vi "Config.vi"() -> ()   [LabVIEW 2010, in "DCP551.lvlib"]
uses:
  DCP551.lvlib
panel:
  in  "Tab Control":T1(tab)
  in  "Read Registers":T2
  in  "Start":bool
  in  "Stop":bool
  in  "Exit":bool
  in  "Server Status":string
  in  "Segment 1 to 99":T3(array[cluster])
  in  "Segment 0":T4={"Start"=enum."Non PV start", "Cycle data"=0, "Pattern link data"=0, "Tag data"="12345678"}
  in  "File ID":string="1"
  in  "Read File":bool
  in  "Write File":bool
  in  "Config":bool
  in  "Serial Config":T5={"串口选择"="COM1", "通讯速率"=9600, "超时时间"=200, "数据位长"=8, "奇偶校验"=enum."Even", "停止位长"=10, "握手控制"=0, "字符结束"=TRUE, "结束字符"=10, "仪器地址"=1} {"结束字符" format="%.0x"; "握手控制" items=["None", "XON/XOFF", "RTS/CTS", "XON/XOFF & RTS/CTS", "DTR/DSR", "XON/XOFF & DTR/DSR"]; "停止位长" items=["1.0"=10, "1.5"=15, "2.0"=20]; "数据位长" min=5 max=8 step=1}
  in  "Write Registers":T6
  in  "RUN":bool
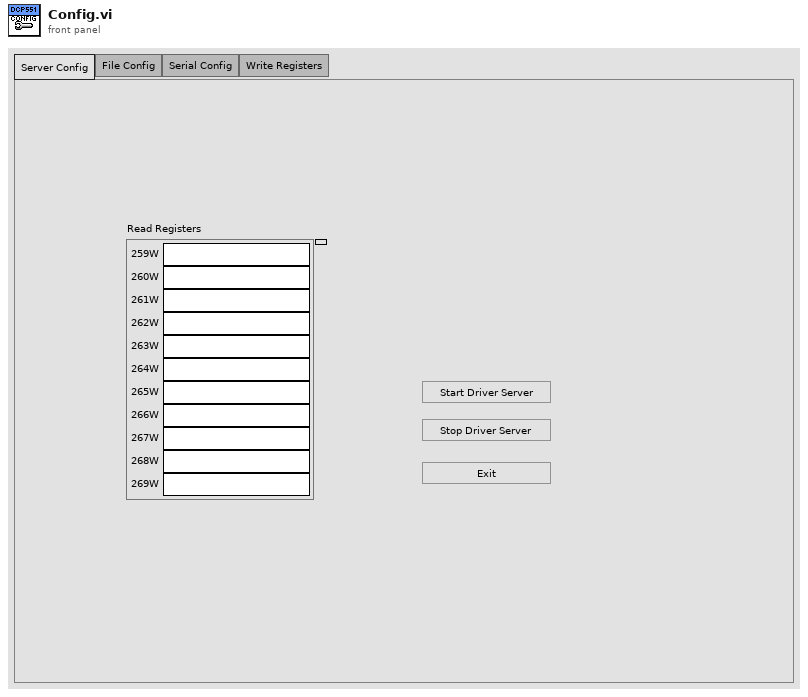
[diagram p1: front panel]
types:
  T1 = enum32{"Server Config", "File Config", "Serial Config", "Write Registers"}
  T2 = cluster{"259W":string, "260W":string, "261W":string, "262W":string, "263W":string, "264W":string, "265W":string, "266W":string, "267W":string, "268W":string, "269W":string}
  T3 = cluster{"SP":dbl, "Time":cluster{"Type":enum16{"Time Data", "delta Dtada", "SP Data"}, "Data":i32}, "EV1 to 16":cluster{"Event 1st data":i32, "Event 2nd data":i32}[], "Output limiter group data":i32, "PID group data":i32, "Repeat return segment data":i32, "Repeat data":i32, "G. soak type data":enum16{"G. soak setting is not provided", "Segment start point", "Segment end point", "Total segment"}, "G. soak width data":i32, "PV shift data":i32}[]
  T4 = cluster{"Start":enum16{"Non PV start", "Upward PV tart", "Downward PV start", "Either upward of downward PV start"}, "Cycle data":i32, "Pattern link data":i32, "Tag data":string}
  T5 = cluster{"串口选择":refnum<visa-resource-name>, "通讯速率":u32, "超时时间":u32, "数据位长":u16, "奇偶校验":enum16{"None", "Odd", "Even", "Mark", "Space"}, "停止位长":u16, "握手控制":u16, "字符结束":bool, "结束字符":u8, "仪器地址":u32}
  T6 = cluster{"261W":string, "262W":string, "263W":string, "264W":string, "265W":string}
  T7 = enum32{"invalid app kind", "Development System", "Run Time System", "Student Edition", "Embedded LabVIEW", "Evaluation", "Custom"}
  T8 = enum32{"Invalid", "Standard", "Closed", "Hidden", "Minimized", "Maximized"}
  T9 = cluster{"Core":cluster{"Current VI Reference":refnum<vi>, "Close Panel on Exit?":bool}, "Your Boolean data":bool, "Your string data":string}
  T10 = cluster{"Current VI Reference":refnum<vi>, "Close Panel on Exit?":bool}
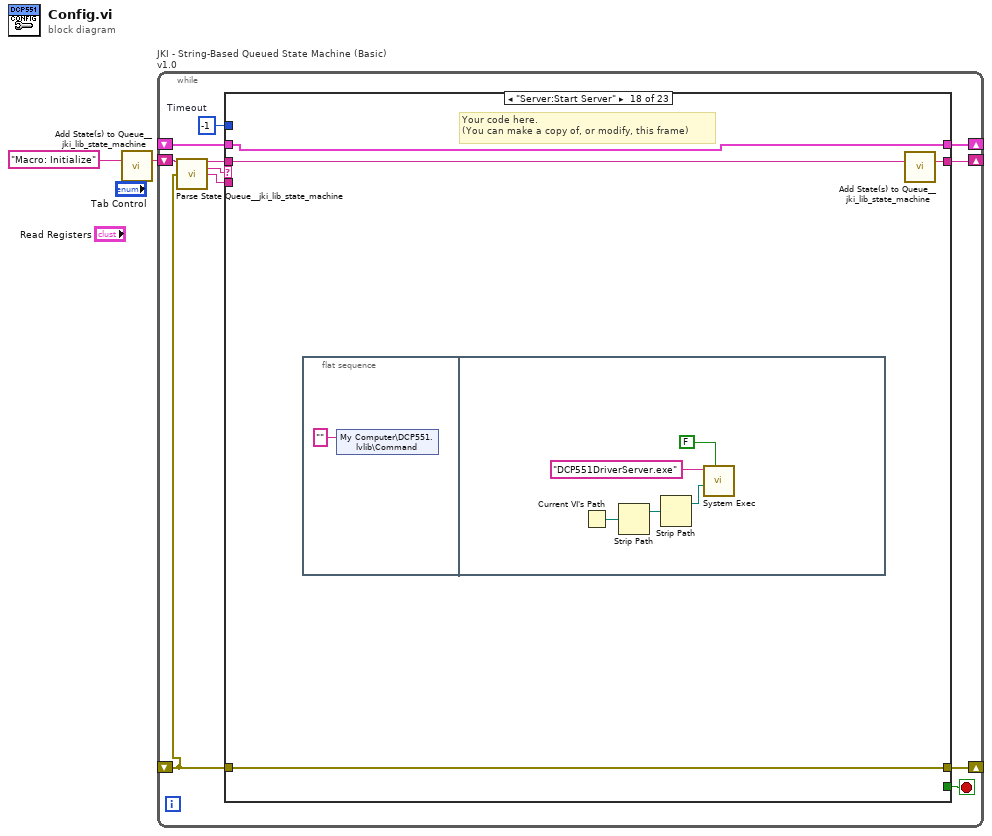
[diagram p0: block diagram]
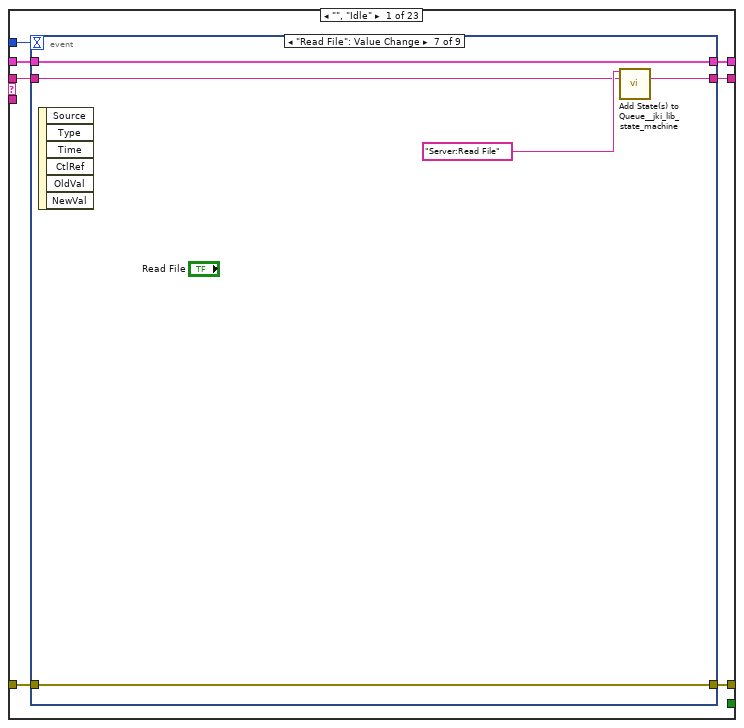
[diagram p2: hidden frame]
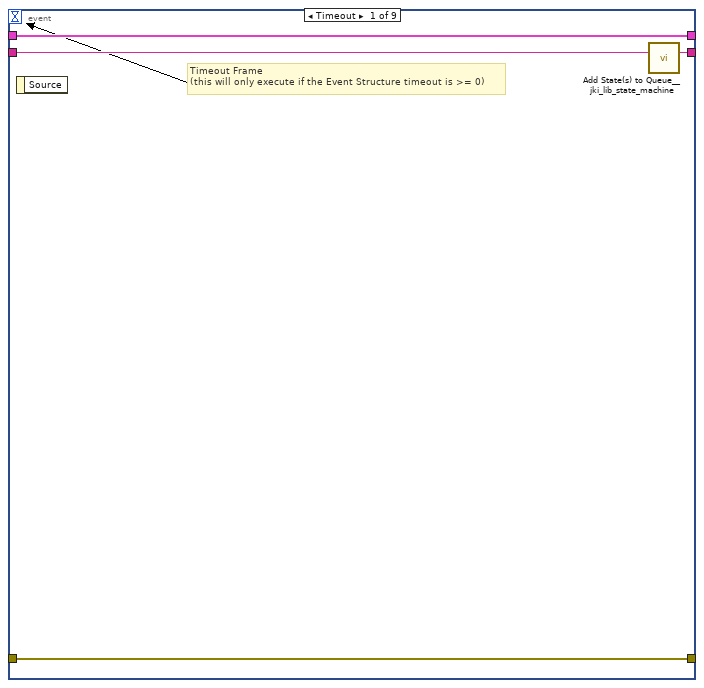
[diagram p3: hidden frame]
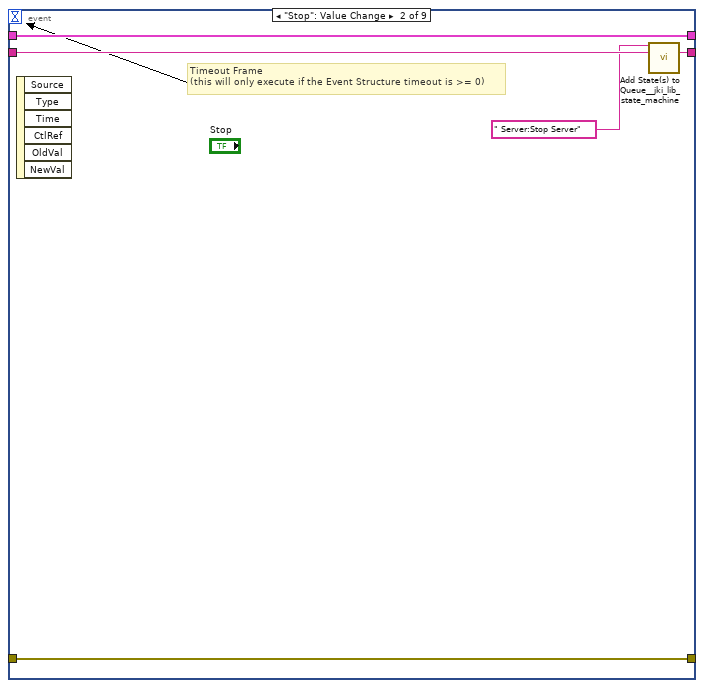
[diagram p4: hidden frame]
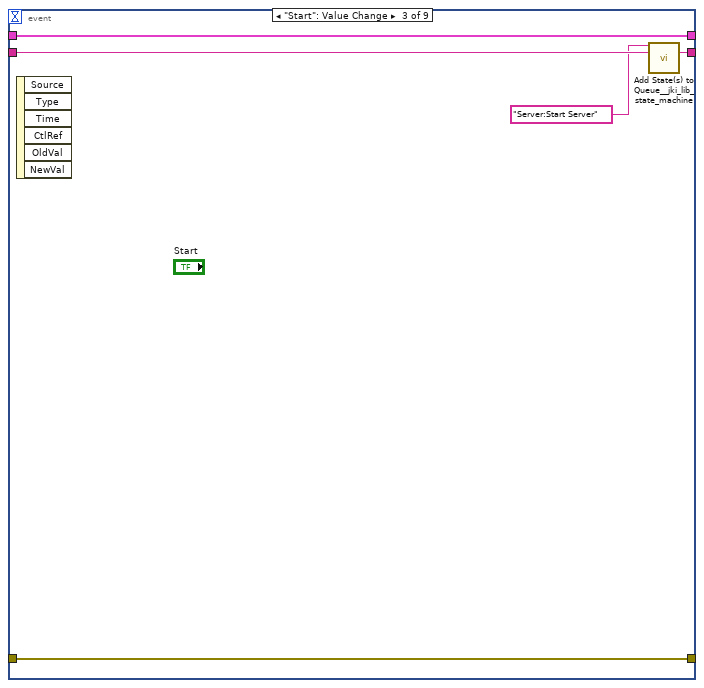
[diagram p5: hidden frame]
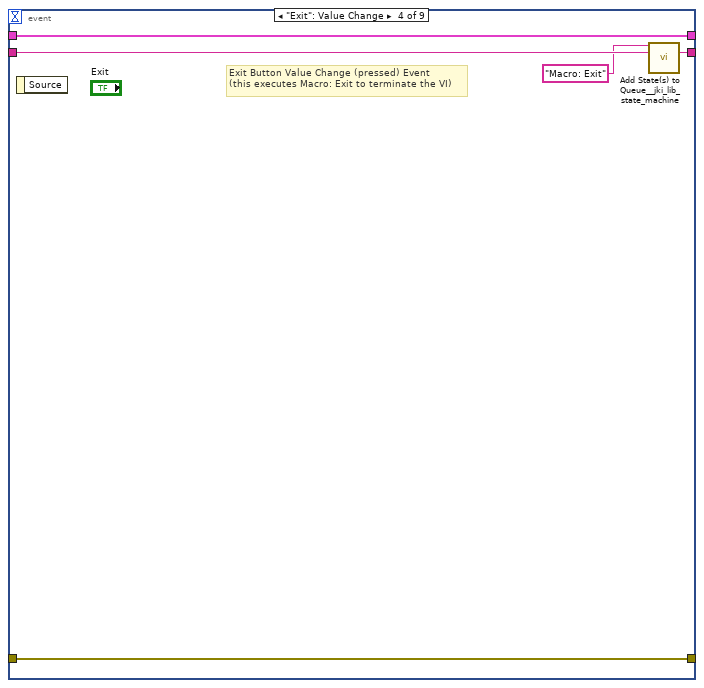
[diagram p6: hidden frame]
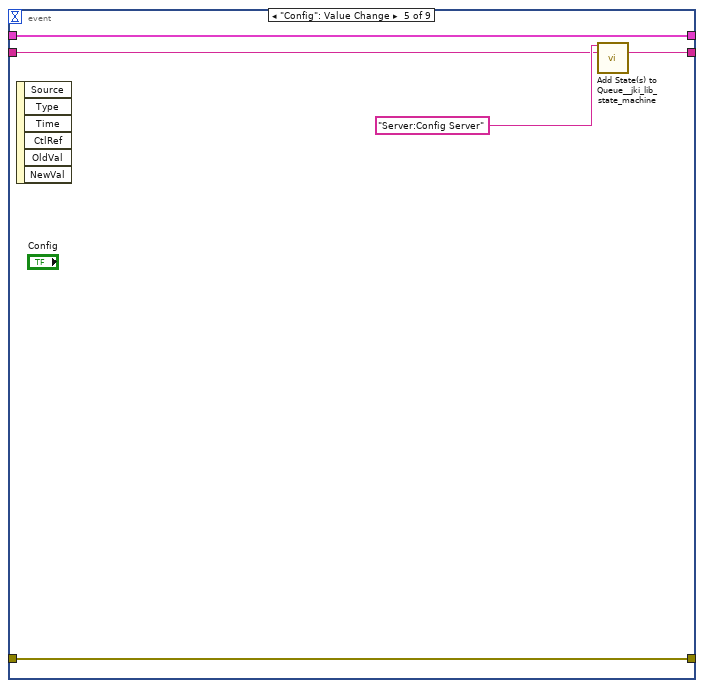
[diagram p7: hidden frame]
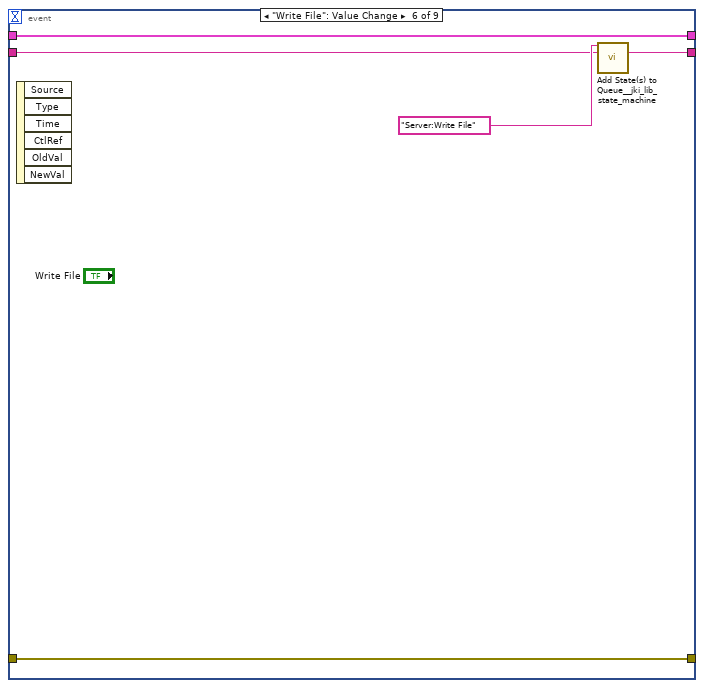
[diagram p8: hidden frame]
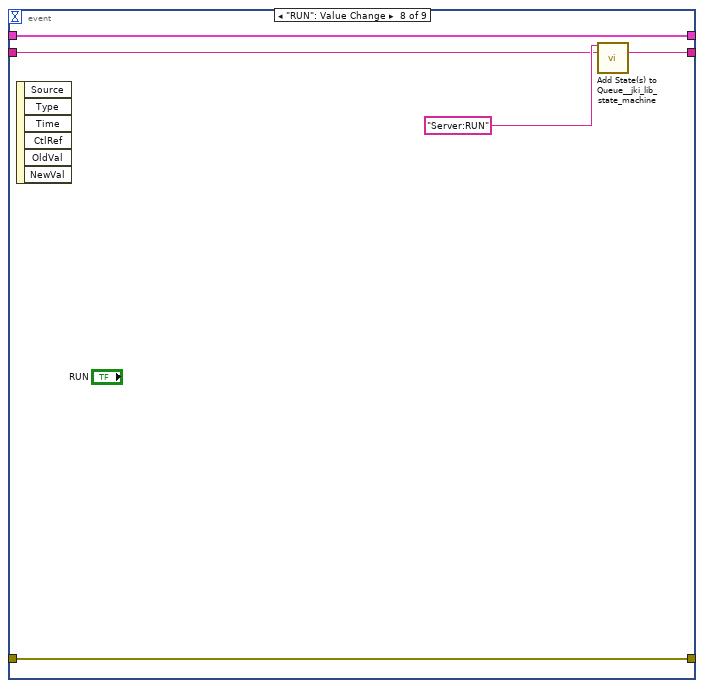
[diagram p9: hidden frame]
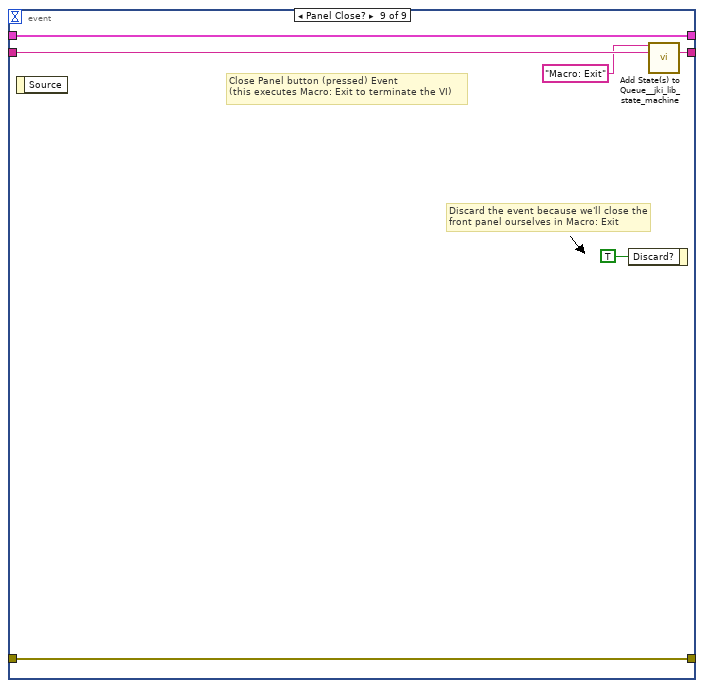
[diagram p10: hidden frame]
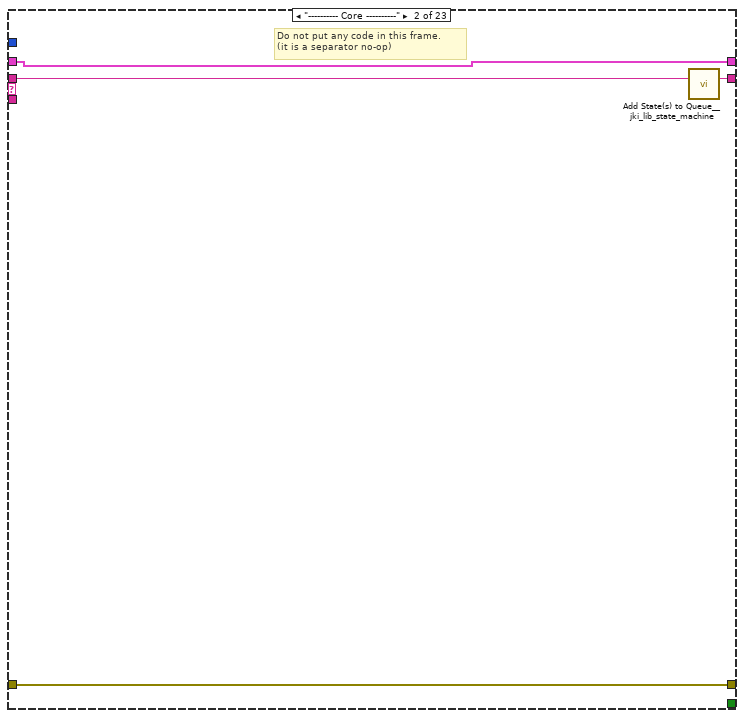
[diagram p11: hidden frame]
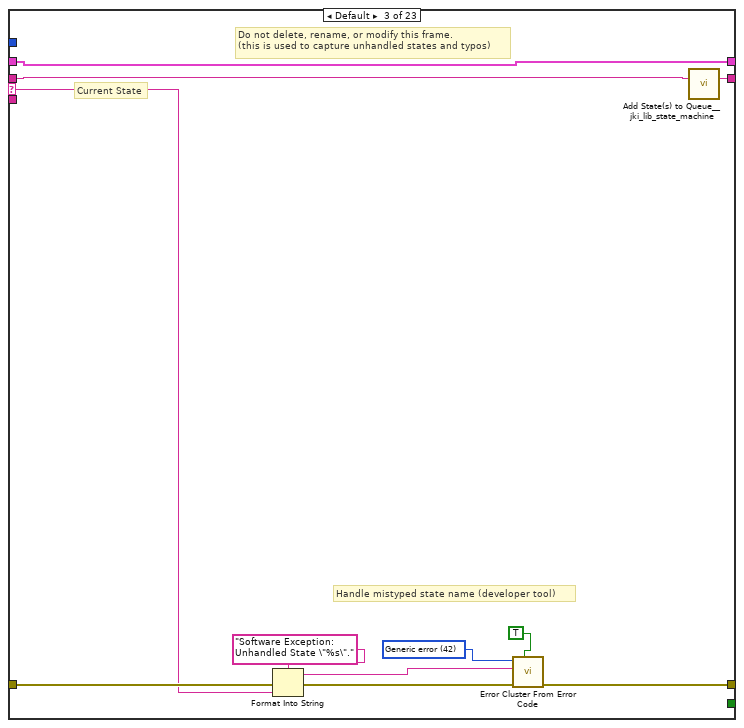
[diagram p12: hidden frame]
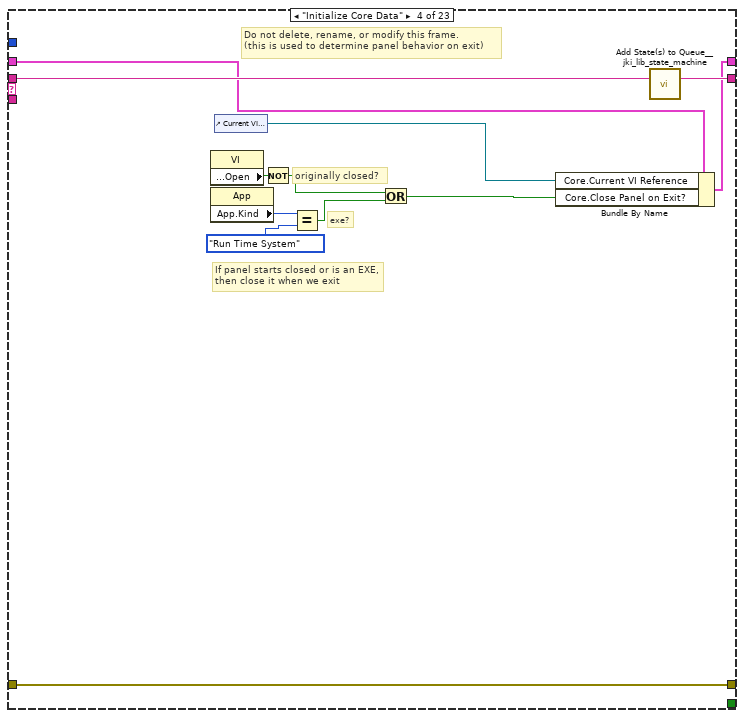
[diagram p13: hidden frame]
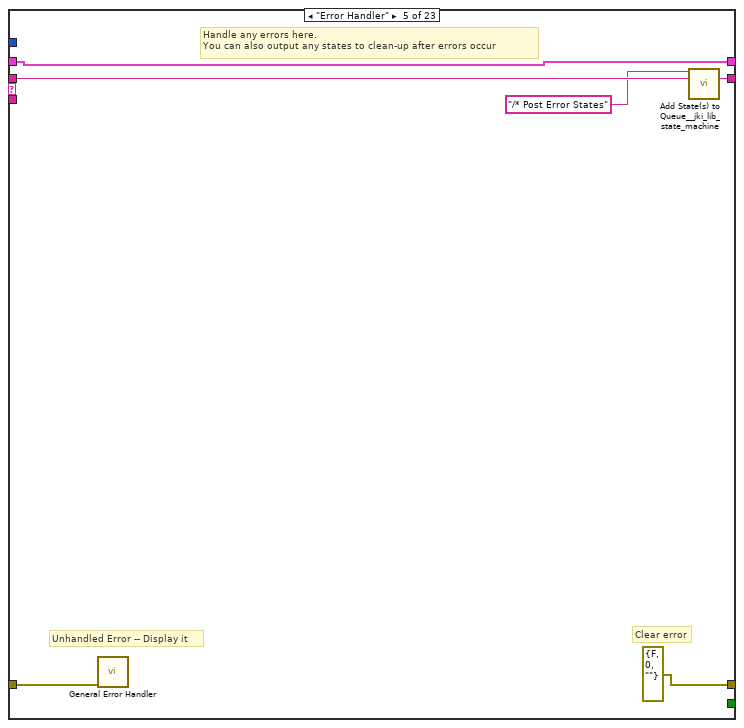
[diagram p14: hidden frame]
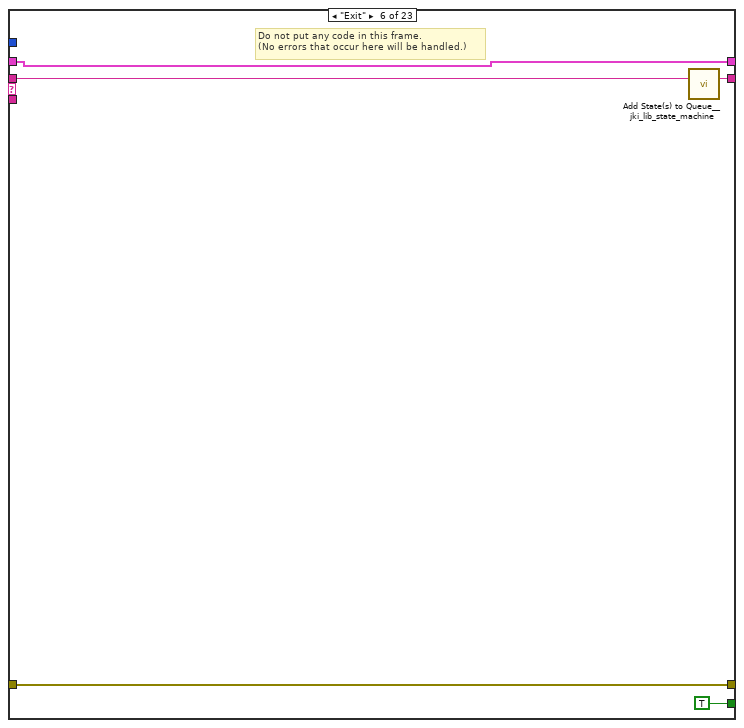
[diagram p15: hidden frame]
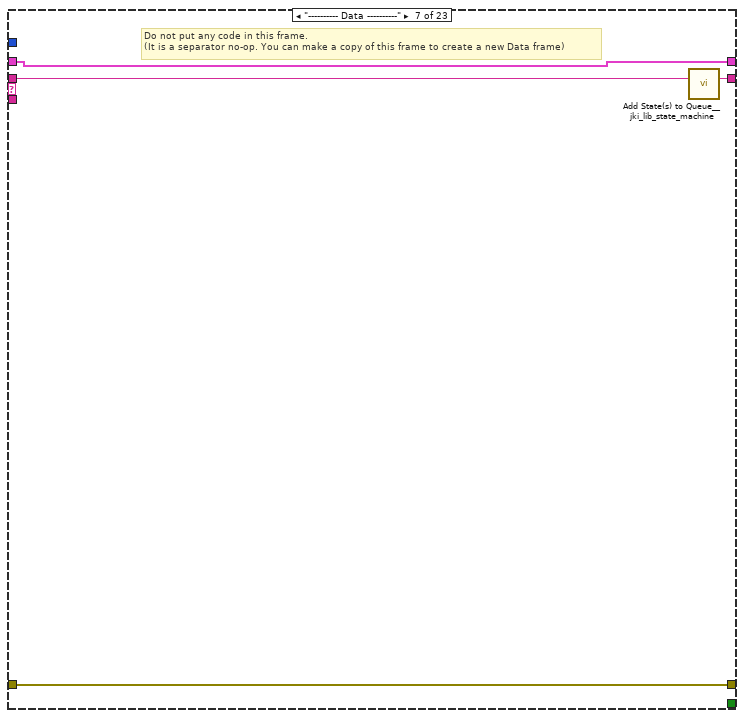
[diagram p16: hidden frame]
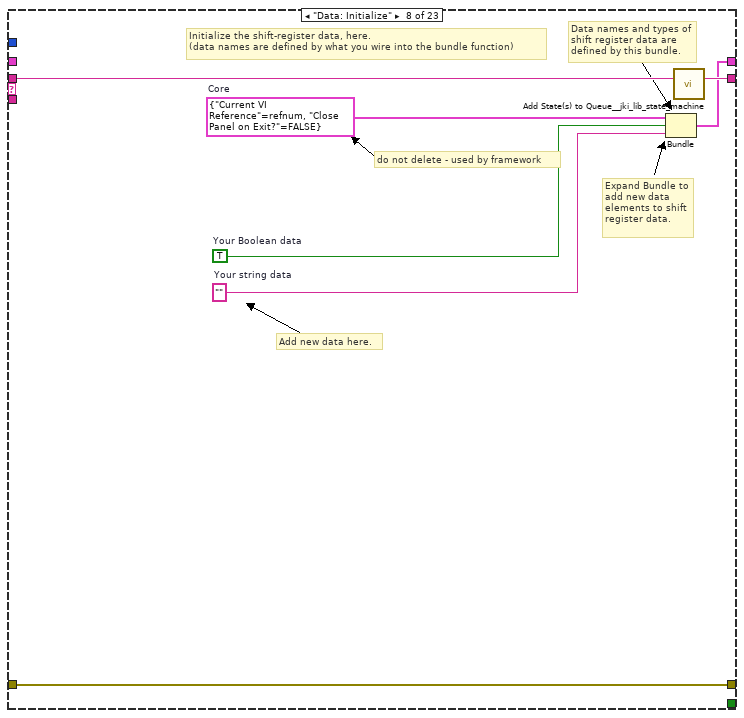
[diagram p17: hidden frame]
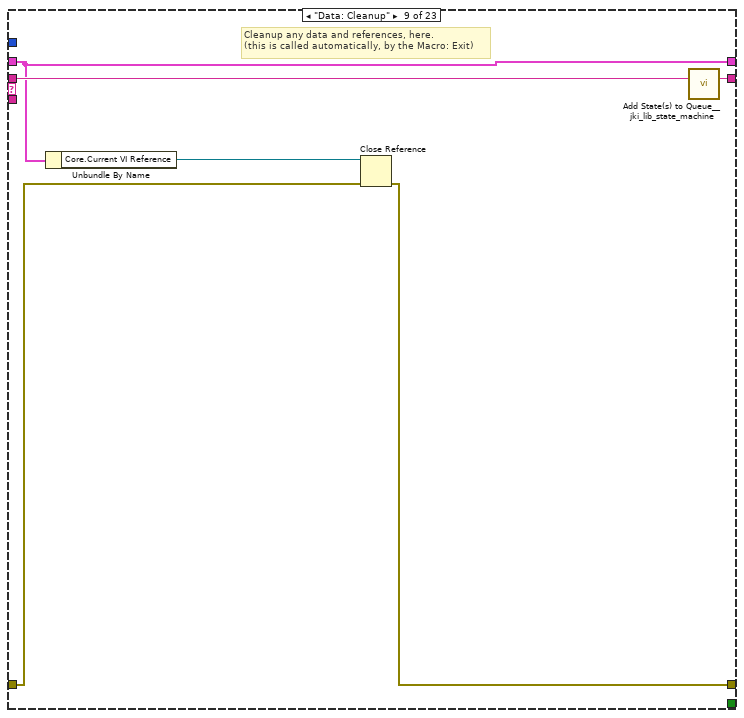
[diagram p18: hidden frame]
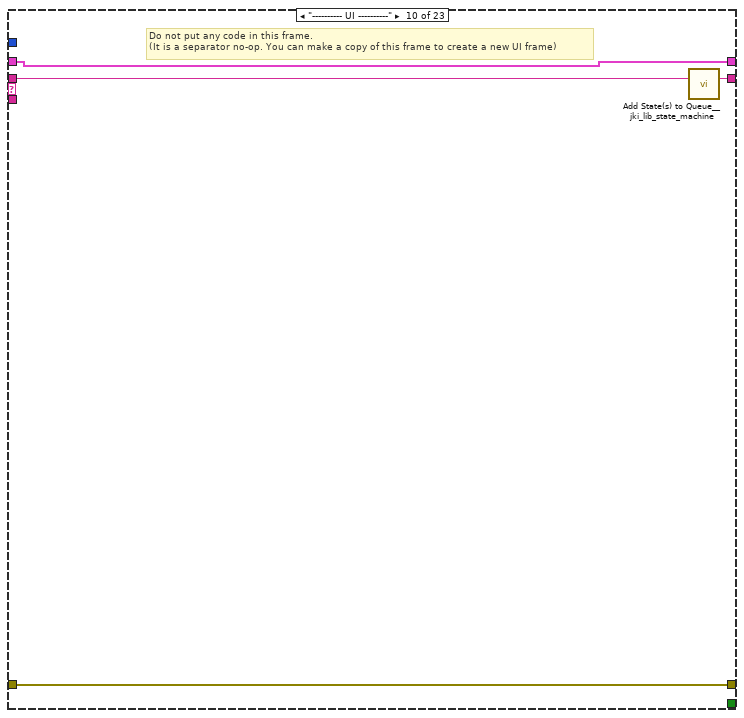
[diagram p19: hidden frame]
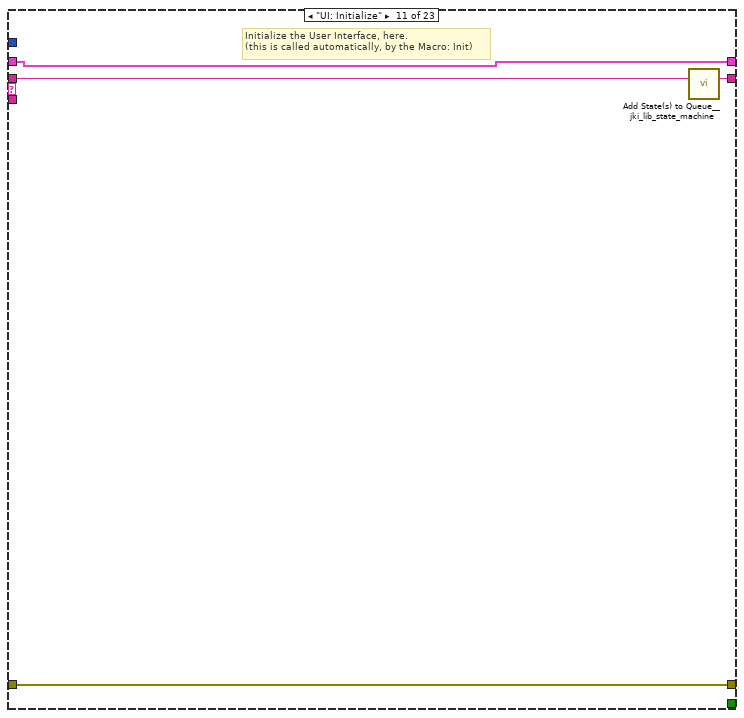
[diagram p20: hidden frame]
diagram:
  n1 = call "Add State(s) to Queue__jki_lib_state_machine.vi"("State(s) in (\"\")"="Macro: Initialize") -> ("States Out"=w2:string)  [unwired: 14 in]
  n2 = while "JKI - String-Based Queued State Machine (Basic) v1.0" {
    shift-right: [w6] -> _
    shift-left: _ -> [w5]
    shift-right: [w9] -> _
    shift-left: _ -> [w3]
    shift-right: [w8] -> _
    shift-left: w2 -> [w10]
    stop <- w7 stop-if-true
    w4 = -1  # Timeout
    n3 = call "Parse State Queue__jki_lib_state_machine.vi"("State Queue"=w10, "Error In (no error)"=w3) -> ("Remaining States"=w12:string, "Current State"=w13:string, "Arguments"=w11:string)  [unwired: 11 in]
    n4 = case shown="\"Server:Start Server\"" w13 {
      selector: w13 -> [_ _ w70 _ _ _ _ _ _ _ _ _ _ _ _ _ _ _ _ _ _ _ _]
      tunnel: w12 -> [w20 w69 w74 w92 w98 w103 w107 w114 w120 w124 w128 w134 w145 w171 w177 w188 w192 w196 w207 w211 w220 w234 w242]
      tunnel: w11 -> [_ _ _ _ _ _ _ _ _ _ _ w129 w139 _ _ _ _ _ _ _ _ _ _]
      tunnel: w5 -> [w18 w66 w72 w83 w95 w101 w104 _ w115 w121 w126 w132 w141 w168 w174 w185 w189 w193 w204 w208 w217 w231 w239]
      tunnel: [w17 w67 w76 w89 errorcluster {"status"=FALSE, "code"=0, "source"=""} ("error out") w100 w105 w111 w116 w122 w125 w130 w142 w169 w175 w186 w190 w194 w205 w209 w218 w232 w240] -> w9
      tunnel: w3 -> [w16 w67 w75 w89 w94 w100 w105 w111 w117 w122 w125 w131 w143 w169 w175 w186 w190 w194 w205 w209 w218 w232 w240]
      tunnel: [w19 w68 w73 w91 w97 w102 w106 w113 w119 w123 w127 w133 w144 w170 w176 w187 w191 w195 w206 w210 w219 w233 w241] -> w8
      tunnel: [_ _ _ _ _ TRUE _ _ _ _ _ _ _ _ _ _ _ _ _ _ _ _ _] -> w7
      tunnel: [w15 w66 w72 w90 w95 w101 w104 w112 w115 w121 w126 w132 w141 w168 w174 w185 w189 w193 w204 w208 w217 w231 w239] -> w6
      tunnel: w4 -> [w14 _ _ _ _ _ _ _ _ _ _ _ _ _ _ _ _ _ _ _ _ _ _]
      frame "", "Idle" {
        n5 = event shown="[6] \"Read File\": Value Change" {
          selector: _ -> [_ _ _ _ _ _ _ _ _]
          dyn-events: _ -> [_ _ _ _ _ _ _ _ _]
          timeout: w14 -> [_ _ _ _ _ _ _ _ _]
          tunnel: w20 -> [w24 w29 w34 w39 w41 w46 w51 w56 w65]
          tunnel: [w23 w28 w33 w38 w40 w45 w50 w55 w64] -> w19
          tunnel: w18 -> [w21 w26 w31 w36 w44 w49 w54 w59 w62]
          tunnel: [w22 w27 w32 w37 w43 w48 w53 w58 w63] -> w17
          tunnel: w16 -> [w22 w27 w32 w37 w43 w48 w53 w58 w63]
          tunnel: [w21 w26 w31 w36 w44 w49 w54 w59 w62] -> w15
          event Timeout {
            # "Timeout Frame\n(this will only execute if the Event Structure timeout is >= 0)"
            n6 = event-data() -> ()  [unwired: 1 in, 1 out]
            n7 = call "Add State(s) to Queue__jki_lib_state_machine.vi"("State(s) in (\"\")"=w24) -> ("States Out"=w23:string)  [unwired: 14 in]
          }
          event "Stop": Value Change {
            # "Timeout Frame\n(this will only execute if the Event Structure timeout is >= 0)"
            n8 = event-data() -> ()  [unwired: 1 in, 6 out]
            n9 = call "Add State(s) to Queue__jki_lib_state_machine.vi"("State(s) in Front (\"\")"=" Server:Stop Server" ("State(s) in Front (\"\")"), "State(s) in (\"\")"=w29) -> ("States Out"=w28:string)  [unwired: 13 in]
          }
          event "Start": Value Change {
            n10 = event-data() -> ()  [unwired: 1 in, 6 out]
            n11 = call "Add State(s) to Queue__jki_lib_state_machine.vi"("State(s) in Front (\"\")"="Server:Start Server" ("State(s) in Front (\"\")"), "State(s) in (\"\")"=w34) -> ("States Out"=w33:string)  [unwired: 13 in]
          }
          event "Exit": Value Change {
            # "Exit Button Value Change (pressed) Event\n(this executes Macro: Exit to terminate the VI)"
            n12 = event-data() -> ()  [unwired: 1 in, 1 out]
            n13 = call "Add State(s) to Queue__jki_lib_state_machine.vi"("State(s) in Front (\"\")"="Macro: Exit", "State(s) in (\"\")"=w39) -> ("States Out"=w38:string)  [unwired: 13 in]
          }
          event "Config": Value Change {
            n14 = event-data() -> ()  [unwired: 1 in, 6 out]
            n15 = call "Add State(s) to Queue__jki_lib_state_machine.vi"("State(s) in Front (\"\")"="Server:Config Server" ("State(s) in Front (\"\")"), "State(s) in (\"\")"=w41) -> ("States Out"=w40:string)  [unwired: 13 in]
          }
          event "Write File": Value Change {
            n16 = event-data() -> ()  [unwired: 1 in, 6 out]
            n17 = call "Add State(s) to Queue__jki_lib_state_machine.vi"("State(s) in Front (\"\")"="Server:Write File" ("State(s) in Front (\"\")"), "State(s) in (\"\")"=w46) -> ("States Out"=w45:string)  [unwired: 13 in]
          }
          event "Read File": Value Change {
            n18 = event-data() -> ()  [unwired: 1 in, 6 out]
            n19 = call "Add State(s) to Queue__jki_lib_state_machine.vi"("State(s) in Front (\"\")"="Server:Read File" ("State(s) in Front (\"\")"), "State(s) in (\"\")"=w51) -> ("States Out"=w50:string)  [unwired: 13 in]
          }
          event "RUN": Value Change {
            n20 = event-data() -> ()  [unwired: 1 in, 6 out]
            n21 = call "Add State(s) to Queue__jki_lib_state_machine.vi"("State(s) in Front (\"\")"="Server:RUN" ("State(s) in Front (\"\")"), "State(s) in (\"\")"=w56) -> ("States Out"=w55:string)  [unwired: 13 in]
          }
          event Panel Close? {
            # "Discard the event because we'll close the front panel ourselves in Macro: Exit"
            # "Close Panel button (pressed) Event\n(this executes Macro: Exit to terminate the VI)"
            n22 = event-data() -> ()  [unwired: 1 in, 1 out]
            n23 = event-data("Discard?"=TRUE) -> ()  [unwired: 1 in, 1 out]
            n24 = call "Add State(s) to Queue__jki_lib_state_machine.vi"("State(s) in Front (\"\")"="Macro: Exit", "State(s) in (\"\")"=w65) -> ("States Out"=w64:string)  [unwired: 13 in]
          }
        }
      }
      frame "---------- Core ----------" {
        # "Do not put any code in this frame.\n(it is a separator no-op)"
        n25 = call "Add State(s) to Queue__jki_lib_state_machine.vi"("State(s) in (\"\")"=w69) -> ("States Out"=w68:string)  [unwired: 14 in]
      }
      frame Default {
        w79 = 42 items=["No error", "Argument error", "Memory is full", "Out of zone", "End of file", "File already open", "Generic file I/O error", "File not found", "File permission error", "Disk is full", "Duplicate path", "Too many files open", "System feature not enabled", "Resource file not found", "Cannot add resource", "Resource not found", "Image not found", "Image memory error", "Pen does not exist", "Config type invalid", "Config token not found", "Config parse error", "Config memory error", "Bad external code format", "Bad external code offset", "External code not present", "Null window", "Destroy window error", "Null menu", "Print aborted", "Bad print record", "Print driver error", "Windows error during printing", "Memory error during printing", "Print dialog error", "Generic print error", "Invalid device refnum", "Device not found", "Device parameter error", "Device unit error", "Cannot open device", "Device call aborted", "Generic error", "Cancelled by user", "Object ID too low", "Object ID too high", "Object not in heap", "Unknown heap", "Unknown object (invalid DefProc)", "Unknown object (DefProc not in table)", "Message out of range", "Invalid (null) method", "Unknown message", "Manager call not supported", "Bad address", "Network operation in progress", "Network operation timed out", "Connection is busy", "Network attribute not supported", "Network error", "Address in use", "System out of memory", "Connection aborted", "Connection refused", "Not connected", "Already connected", "Connection closed", "Initialization error (interapplication manager)", "Bad occurrence", "Wait on unbound occurrence handler", "Occurrence queue overflow", "Datalog type conflict", "Unused", "Unrecognized type (interapplication manager)", "Memory corrupt", "Failed to make temporary DLL", "Old CIN version", "Drag socket not found", "Failed to load drop-object", "Failed to register OLE object", "Failed to release OLE object", "Format specifier type mismatch", "Unknown format specifier", "Too few format specifiers", "Too many format specifiers", "Scan failed", "Newer CIN version", "Error converting to variant", "Runtime menu error", "Password tampered", "Variant attribute not found", "Incompatible variant data type", "Event data is not available", "Event Store is not present", "Occurrence is not found", "Event Queue is not created", "Event info is not available", "Refnum passed is NULL", "Error retrieving Class GUID", "Error retrieving CoClass GUID", "Error retrieving TypeLib GUID.", "Bad built application magic bytes.", "Specific driver is different from the specific driver associated with the Logical Name.", "There is no session opened to the class driver.", "Max Error", "MAX - Error with config objects", "MAX - Error loading configuration", "MAX - Group not supported"]
        # "Current State"
        # "Do not delete, rename, or modify this frame.\n(this is used to capture unhandled states and typos)"
        # "Handle mistyped state name (developer tool)"
        n26 = Format Into String(format string="Software Exception: Unhandled State \"%s\"." ("message"), error in=w75, w70) -> (resulting string=w78:string, error out=w77:errorcluster)  [unwired: 1 in]
        n27 = call <vilib>:"Error Cluster From Error Code.vi"("show call chain? (False)"=TRUE, "error in (no error)"=w77, "error message (\"\")"=w78, "error code (0)"=w79) -> ("error out"=w76:errorcluster)  [unwired: 5 in]
        n28 = call "Add State(s) to Queue__jki_lib_state_machine.vi"("State(s) in (\"\")"=w74) -> ("States Out"=w73:string)  [unwired: 14 in]
      }
      frame "Initialize Core Data" {
        # "Do not delete, rename, or modify this frame.\n(this is used to determine panel behavior on exit)"
        # "originally closed?"
        # "exe?"
        # "If panel starts closed or is an EXE, then close it when we exit"
        n29 = property class="VI"() -> ("Front Panel.Open"=w88:bool)  [unwired: 2 in, 2 out]
        n30 = property class="App"() -> ("App.Kind"=w87:T7)  [unwired: 2 in, 2 out]
        n31 = control-ref of="Current VI Reference"() -> (w81:refnum<vi>)
        n32 = Not(x=w88) -> (.not. x?=w85:bool)
        n33 = Equal?(x=w87, y=T7."Run Time System" ("Application:Kind")) -> (x = y?=w84:bool)
        n34 = Or(x=w85, y=w84) -> (x .or. y?=w82:bool)
        n35 = Bundle By Name(cluster=w83, "Core.Current VI Reference"=w81, "Core.Close Panel on Exit?"=w82) -> (w90:T9)
        n36 = call "Add State(s) to Queue__jki_lib_state_machine.vi"("State(s) in (\"\")"=w92) -> ("States Out"=w91:string)  [unwired: 14 in]
      }
      frame "Error Handler" {
        # "Unhandled Error -- Display it"
        # "Handle any errors here.\nYou can also output any states to clean-up after errors occur"
        # "Clear error"
        n37 = call <vilib>:"General Error Handler.vi"("error in (no error)"=w94) -> ()  [unwired: 10 in, 5 out]
        n38 = call "Add State(s) to Queue__jki_lib_state_machine.vi"("State(s) in Front (\"\")"="/* Post Error States", "State(s) in (\"\")"=w98) -> ("States Out"=w97:string)  [unwired: 13 in]
      }
      frame "Exit" {
        # "Do not put any code in this frame.\n(No errors that occur here will be handled.)"
        n39 = call "Add State(s) to Queue__jki_lib_state_machine.vi"("State(s) in (\"\")"=w103) -> ("States Out"=w102:string)  [unwired: 14 in]
      }
      frame "---------- Data ----------" {
        # "Do not put any code in this frame.\n(It is a separator no-op. You can make a copy of this frame to create a new Data frame)"
        n40 = call "Add State(s) to Queue__jki_lib_state_machine.vi"("State(s) in (\"\")"=w107) -> ("States Out"=w106:string)  [unwired: 14 in]
      }
      frame "Data: Initialize" {
        w108 = T10 {"Current VI Reference"=refnum, "Close Panel on Exit?"=FALSE}  # Core
        w110 = TRUE  # Your Boolean data
        w109 = ""  # Your string data
        # "do not delete - used by framework"
        # "Expand Bundle to add new data elements to shift register data."
        # "Add new data here."
        # "Data names and types of shift register data are defined by this bundle."
        # "Initialize the shift-register data, here.\n(data names are defined by what you wire into the bundle function)"
        n41 = Bundle("Core"=w108, "Your Boolean data"=w110, "Your string data"=w109) -> (w112:T9)  [unwired: 1 in]
        n42 = call "Add State(s) to Queue__jki_lib_state_machine.vi"("State(s) in (\"\")"=w114) -> ("States Out"=w113:string)  [unwired: 14 in]
      }
      frame "Data: Cleanup" {
        # "Cleanup any data and references, here.\n(this is called automatically, by the Macro: Exit)"
        n43 = Unbundle By Name(w115) -> ("Core.Current VI Reference"=w118:refnum<vi>)
        n44 = Close Reference(reference=w118, error in (no error)=w117) -> (error out=w116:errorcluster)
        n45 = call "Add State(s) to Queue__jki_lib_state_machine.vi"("State(s) in (\"\")"=w120) -> ("States Out"=w119:string)  [unwired: 14 in]
      }
      frame "---------- UI ----------" {
        # "Do not put any code in this frame.\n(It is a separator no-op. You can make a copy of this frame to create a new UI frame)"
        n46 = call "Add State(s) to Queue__jki_lib_state_machine.vi"("State(s) in (\"\")"=w124) -> ("States Out"=w123:string)  [unwired: 14 in]
      }
      frame "UI: Initialize" {
        # "Initialize the User Interface, here.\n(this is called automatically, by the Macro: Init)"
        n47 = call "Add State(s) to Queue__jki_lib_state_machine.vi"("State(s) in (\"\")"=w128) -> ("States Out"=w127:string)  [unwired: 14 in]
      }
      frame "UI: Cursor Set" {
        # "Argument"
        # "Set and Unset Cursor Busy.\n(Usage: \"UI: Cursor Set >> Busy|Idle\")"
        n48 = case shown="\"Idle\", Default" w129 {
          tunnel: w131 -> [w136 w138]
          tunnel: [w135 w137] -> w130
          frame "Idle", Default {
            n49 = call <vilib>:"Unset Busy.vi"("error in (no error)"=w136) -> ("error out"=w135:errorcluster)  [unwired: 10 in]
          }
          frame "Busy" {
            n50 = call <vilib>:"Set Busy.vi"("error in (no error)"=w138) -> ("error out"=w137:errorcluster)  [unwired: 9 in, 1 out]
          }
        }
        n51 = call "Add State(s) to Queue__jki_lib_state_machine.vi"("State(s) in (\"\")"=w134) -> ("States Out"=w133:string)  [unwired: 14 in]
      }
      frame "UI: Front Panel State" {
        # "Argument"
        # "Set Front Panel Open or Closed\n(Usage: \"UI: Front Panel State >> Open|Close\")"
        n52 = Unbundle By Name(w141) -> ("Core.Current VI Reference"=w140:refnum<vi>)
        n53 = case shown="\"Open\", Default" w139 {
          tunnel: w143 -> [w149 w162]
          tunnel: [w151 w163] -> w142
          tunnel: w140 -> [w150 w160]
          frame "Open", Default {
            n54 = property class="VI"(reference=w150, error in=w149) -> (reference out=w147:refnum<vi>, error out=w148:errorcluster, "Front Panel.Open"=w146:bool)
            n55 = case shown="True" w146 {
              tunnel: [w154 w157] -> w151
              tunnel: w148 -> [w153 w157]
              tunnel: w147 -> [w152 _]
              frame False {
                n56 = invoke class="VI" method="FP.Open"(reference=w152, error in=w153, "Activate"=TRUE, "State"=T8."Standard") -> (error out=w154:errorcluster)  [unwired: 1 in, 4 out]
              }
              frame True {
              }
            }
          }
          frame "Close" {
            n57 = property class="VI"(reference=w160, error in=w162) -> (reference out=w159:refnum<vi>, error out=w161:errorcluster, "Front Panel.Open"=w158:bool)
            n58 = case shown="True" w158 {
              tunnel: [w164 w167] -> w163
              tunnel: w161 -> [w164 w166]
              tunnel: w159 -> [_ w165]
              frame False {
              }
              frame True {
                n59 = invoke class="VI" method="FP.Close"(reference=w165, error in=w166) -> (error out=w167:errorcluster)  [unwired: 1 in, 2 out]
              }
            }
          }
        }
        n60 = call "Add State(s) to Queue__jki_lib_state_machine.vi"("State(s) in (\"\")"=w145) -> ("States Out"=w144:string)  [unwired: 14 in]
      }
      frame "---------- Macro ----------" {
        # "Do not put any code in this frame.\n(It is a separator no-op. You can make a copy of this frame to create a new Macro frame)"
        n61 = call "Add State(s) to Queue__jki_lib_state_machine.vi"("State(s) in (\"\")"=w171) -> ("States Out"=w170:string)  [unwired: 14 in]
      }
      frame "Macro: Initialize" {
        w173 = "Data: Initialize\nInitialize Core Data\nUI: Initialize\nUI: Front Panel State >> Open"  # Data: Initialize Initialize Core Data UI: Initialize UI: Front Panel State >> Open
        # "Initialization Macro\n(This is called once, when the VI starts)"
        n62 = shared-variable "My Computer\\DCP551.lvlib\\Server Status"("Working" ("Server Status")) -> ()  [unwired: 1 in, 1 out]
        n63 = call "Add State(s) to Queue__jki_lib_state_machine.vi"("State(s) in Front (\"\")"=w173, "State(s) in (\"\")"=w177) -> ("States Out"=w176:string)  [unwired: 13 in]
      }
      frame "Macro: Exit" {
        n64 = Unbundle By Name(w185) -> ("Core.Close Panel on Exit?"=w184:bool)
        n65 = shared-variable "My Computer\\DCP551.lvlib\\Server Status"("Stopped" ("Server Status")) -> ()  [unwired: 1 in, 1 out]
        n66 = Select(t="UI: Front Panel State >> Close", s=w184, f="") -> (s? t:f=w181:string)
        n67 = call "Add State(s) to Queue__jki_lib_state_machine.vi"("State(s) in (\"\")"=w181, "State(s) at Back (\"\")"="Data: Cleanup\nExit") -> ("States Out"=w179:string)  [unwired: 13 in]
        n68 = call "Add State(s) to Queue__jki_lib_state_machine.vi"("State(s) in Front (\"\")"=w179, "State(s) in (\"\")"=w188) -> ("States Out"=w187:string)  [unwired: 13 in]
      }
      frame "---------- Server ----------" {
        # "Template Separator\n(You can make a copy of, or modify, this frame)"
        n69 = call "Add State(s) to Queue__jki_lib_state_machine.vi"("State(s) in (\"\")"=w192) -> ("States Out"=w191:string)  [unwired: 14 in]
      }
      frame "Server:Start Server" {
        # "Your code here.\n(You can make a copy of, or modify, this frame)"
        n70 = flat-sequence {
          frame #0 {
            n71 = shared-variable "My Computer\\DCP551.lvlib\\Command"("" ("Command")) -> ()  [unwired: 1 in, 1 out]
          }
          frame #1 {
            n72 = Current VI's Path() -> (path=w202:path)
            n73 = Strip Path(path=w202) -> (stripped path=w201:path)  [unwired: 1 out]
            n74 = Strip Path(path=w201) -> (stripped path=w200:path)  [unwired: 1 out]
            n75 = call <vilib>:"System Exec.vi"("wait until completion? (T)"=FALSE, "working directory"=w200, "command line"="DCP551DriverServer.exe" ("name or relative path")) -> ()  [unwired: 5 in, 4 out]
          }
        }
        n76 = call "Add State(s) to Queue__jki_lib_state_machine.vi"("State(s) in (\"\")"=w196) -> ("States Out"=w195:string)  [unwired: 14 in]
      }
      frame "Server:Stop Server" {
        # "Your code here.\n(You can make a copy of, or modify, this frame)"
        n77 = shared-variable "My Computer\\DCP551.lvlib\\Command"("Macro: Exit" ("Command")) -> ()  [unwired: 1 in, 1 out]
        n78 = call "Add State(s) to Queue__jki_lib_state_machine.vi"("State(s) in (\"\")"=w207) -> ("States Out"=w206:string)  [unwired: 14 in]
      }
      frame "Server:Write File" {
        # "Your code here.\n(You can make a copy of, or modify, this frame)"
        n79 = flat-sequence {
          frame #0 {
            n80 = shared-variable "My Computer\\DCP551.lvlib\\Segment0"("Segment 0") -> ()  [unwired: 1 in, 1 out]
            n81 = shared-variable "My Computer\\DCP551.lvlib\\File ID"("File ID") -> ()  [unwired: 1 in, 1 out]
            n82 = shared-variable "My Computer\\DCP551.lvlib\\Segment 1 to 99"("Segment 1 to 99") -> ()  [unwired: 1 in, 1 out]
          }
          frame #1 {
            n83 = shared-variable "My Computer\\DCP551.lvlib\\Server Status"("Writting" ("Server Status")) -> ()  [unwired: 1 in, 1 out]
            n84 = shared-variable "My Computer\\DCP551.lvlib\\Command"("File:Write" ("Command")) -> ()  [unwired: 1 in, 1 out]
          }
        }
        n85 = call "Add State(s) to Queue__jki_lib_state_machine.vi"("State(s) in (\"\")"=w211) -> ("States Out"=w210:string)  [unwired: 14 in]
      }
      frame "Server:Read File" {
        # "Your code here.\n(You can make a copy of, or modify, this frame)"
        n86 = stacked-sequence {
          frame #0 {
            n87 = property on="File ID" class="Str"() -> ("Value"=w222:string)  [unwired: 2 in, 2 out]
            n88 = shared-variable "My Computer\\DCP551.lvlib\\Server Status"("Reading" ("Server Status")) -> ()  [unwired: 1 in, 1 out]
            n89 = shared-variable "My Computer\\DCP551.lvlib\\File ID"(w222) -> ()  [unwired: 1 in, 1 out]
          }
          frame #1 {
            n90 = shared-variable "My Computer\\DCP551.lvlib\\Command"("File:Read" ("Command")) -> ()  [unwired: 1 in, 1 out]
          }
          frame #2 {
            n91 = while {
              stop <- w225 stop-if-true
              n92 = shared-variable "My Computer\\DCP551.lvlib\\Server Status"() -> (w227:string)  [unwired: 1 in, 1 out]
              n93 = Wait (ms)(milliseconds to wait=u32 100) -> ()  [unwired: 1 out]
              n94 = Equal?(x=w227, y="Read Over") -> (x = y?=w225:bool)
            }
          }
          frame #3 {
            n95 = shared-variable "My Computer\\DCP551.lvlib\\Server Status"("Working" ("Server Status")) -> ()  [unwired: 1 in, 1 out]
          }
          frame #4 {
            n96 = shared-variable "My Computer\\DCP551.lvlib\\Segment 1 to 99"() -> (w229:T3)  [unwired: 1 in, 1 out]
            n97 = shared-variable "My Computer\\DCP551.lvlib\\Segment0"() -> (w230:T4)  [unwired: 1 in, 1 out]
            n98 = property on="Segment 1 to 99" class="Arr (strict)"("Value"=w229) -> ()  [unwired: 2 in, 2 out]
            n99 = property on="Segment 0" class="Clust (strict)"("Value"=w230) -> ()  [unwired: 2 in, 2 out]
          }
        }
        n100 = call "Add State(s) to Queue__jki_lib_state_machine.vi"("State(s) in (\"\")"=w220) -> ("States Out"=w219:string)  [unwired: 14 in]
      }
      frame "Server:RUN" {
        # "Your code here.\n(You can make a copy of, or modify, this frame)"
        n101 = flat-sequence {
          frame #0 {
            n102 = shared-variable "My Computer\\DCP551.lvlib\\Write Registers"("Write Registers") -> ()  [unwired: 1 in, 1 out]
          }
          frame #1 {
            n103 = shared-variable "My Computer\\DCP551.lvlib\\Command"("Register:Write" ("Command")) -> ()  [unwired: 1 in, 1 out]
          }
        }
        n104 = call "Add State(s) to Queue__jki_lib_state_machine.vi"("State(s) in (\"\")"=w234) -> ("States Out"=w233:string)  [unwired: 14 in]
      }
      frame "Server:Config Server" {
        # "Your code here.\n(You can make a copy of, or modify, this frame)"
        n105 = call "Save Config.vi"("FileName"="DCP551SerialConfig.xml", "Serial Config"="Serial Config") -> ()  [unwired: 9 in, 1 out]
        n106 = call "Add State(s) to Queue__jki_lib_state_machine.vi"("State(s) in (\"\")"=w242) -> ("States Out"=w241:string)  [unwired: 14 in]
      }
    }
  }
